vi "IsValid.vi"(8 "error in (no error)":errorcluster, 11 "Plot ID":T1 format="%x") -> (0 "error out":errorcluster, 2 "Valid?":bool, 3 "Plot ID Out":T1 format="%x")   [LabVIEW 2013, in "Advanced Plotting Toolkit.lvlib"]
doc: "Test a plot identifier to see if it's valid."
uses:
  Advanced Plotting Toolkit.lvlib
  typedefs/PlotID.ctl
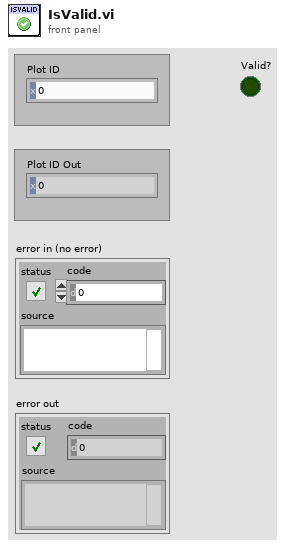
[diagram p1: front panel]
types:
  T1 = typedef "Advanced Plotting Toolkit.lvlib/PlotID.ctl" = i32
  T2 = typedef "Advanced Plotting Toolkit.lvlib/KeyValue.ctl" = cluster{"Key":string, "Value":string}
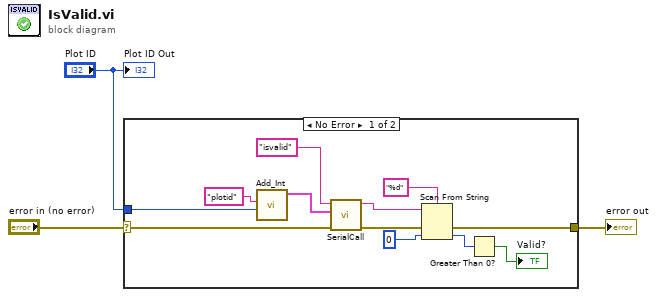
[diagram p0: block diagram]
diagram:
  n1 = case shown="No Error" "error in (no error)" {
    selector: "error in (no error)" -> [w11 w16]
    tunnel: [w9 w16] -> w3
    tunnel: "Plot ID" -> [w12 _]
    frame No Error {
      n2 = call "Add_Int.vi"("Value"=w12, "Key"="plotid") -> ("Keyword Array Out"=w13:T2[])  [unwired: 9 in]
      n3 = call "SerialCall.vi"("error in (no error)"=w11, "data"=w13, "Resource"="isvalid") -> ("error out"=w10:errorcluster, "Response"=w8:string)  [unwired: 7 in]
      n4 = Scan From String(format string="%d", input string=w8, error in=w10, default 1=0 ("default value 1")) -> (error out=w9:errorcluster, output 1=w6:i32)  [unwired: 1 in, 2 out]
      n5 = Greater Than 0?(x=w6) -> (x > 0?=→"Valid?":bool)
    }
    frame Error {
    }
  }
  "error out" <- w3
  "Plot ID Out" <- "Plot ID"
